vi "Init Hardware.vi"(8 "error in (no error)":errorcluster, 11 "Micron sm Digitizer in":refnum<class "Micron sm Digitizer.lvclass">) -> (0 "error out":errorcluster, 3 "Micron sm Digitizer out":refnum<class "Micron sm Digitizer.lvclass">)   [LabVIEW 2024, in "Micron sm Digitizer.lvclass"]
uses:
  Micron sm Digitizer.lvclass
  C:/Git/NHMFL_Core/Libraries/Instruments/VISA Instrument/VISA Instrument.lvclass
  C:/Git/NHMFL_Core/Libraries/Instruments/Instrument Driver/Instrument Driver.lvclass
  VISA Instrument/VISA Instrument.lvclass/VISA Instrument.ctl
  Instrument Driver/Instrument Driver.lvclass/Instrument Driver.ctl
  VISA Instrument/Read VISA resource.vi
  Instrument Driver/Read Cycle period.vi
  VISA Instrument/Write VISA resource.vi
  Micron Optics sm130/Micron Optics sm130.lvlib
panel:
  out "Rate":i32
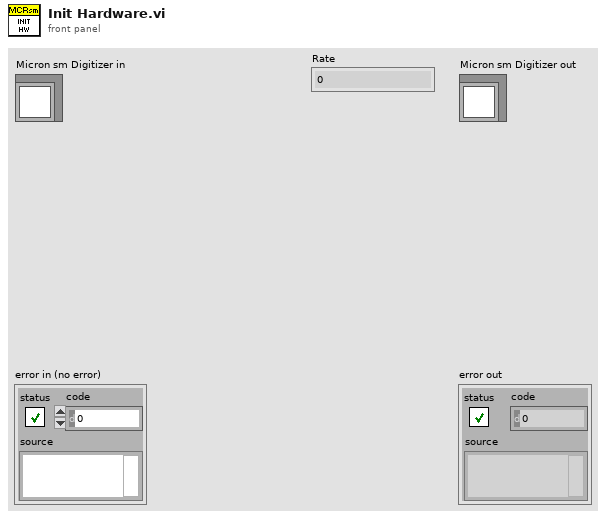
[diagram p1: front panel]
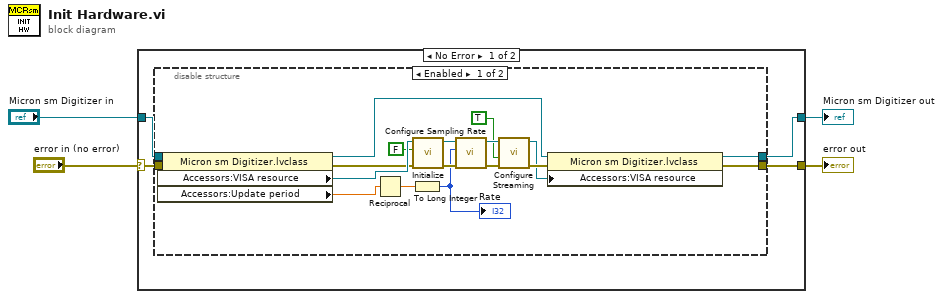
[diagram p0: block diagram]
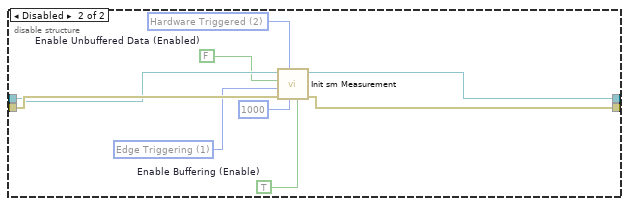
[diagram p2: hidden frame]
diagram:
  n1 = case shown="No Error" "error in (no error)" {
    selector: "error in (no error)" -> [w5 w36]
    tunnel: "Micron sm Digitizer in" -> [w8 w37]
    tunnel: [w7 w36] -> w3
    tunnel: [w6 w37] -> w2
    frame No Error {
      n2 = disable-structure shown="Enabled" {
        disable-tunnel: w8 -> [w26 w33]
        disable-tunnel: [w12 w34] -> w7
        disable-tunnel: [w11 w32] -> w6
        disable-tunnel: w5 -> [w10 w35]
        frame Enabled {
          n3 = property class="Micron sm Digitizer.lvclass"(reference=w26, error in=w10) -> (reference out=w15:refnum<class "Micron sm Digitizer.lvclass">, error out=w24:errorcluster, "Accessors:VISA resource"=w25:refnum<visa-resource-name>, "Accessors:Update period"=w21:dbl)
          n4 = Reciprocal(x=w21) -> (1/x=w20:dbl)
          n5 = To Long Integer(number=w20) -> (32bit integer=w19:i32)
          "Rate" <- w19
          n6 = call "Initialize.vi"("error in (no error)"=w24, "ID Query (True)"=FALSE, "VISA resource name"=w25) -> ("error out"=w23:errorcluster, "VISA resource name out"=w22:refnum<visa-resource-name>)  [unwired: 7 in]
          n7 = call "Configure Sampling Rate.vi"("error in (no error)"=w23, "Sample Rate (1000 Hz)"=w19, "VISA resource name"=w22) -> ("error out"=w17:errorcluster, "VISA resource name out"=w18:refnum<visa-resource-name>)  [unwired: 7 in]
          n8 = call "Configure Streaming.vi"("error in (no error)"=w17, "Enable Streaming (Enable)"=TRUE, "VISA resource name"=w18) -> ("error out"=w14:errorcluster, "VISA resource name out"=w13:refnum<visa-resource-name>)  [unwired: 7 in]
          n9 = property class="Micron sm Digitizer.lvclass"(reference=w15, error in=w14, "Accessors:VISA resource"=w13) -> (reference out=w11:refnum<class "Micron sm Digitizer.lvclass">, error out=w12:errorcluster)
        }
        frame Disabled {
          w28 = u16 2 items=["Untriggered", "Software Triggered", "Hardware Triggered"] ("Trigger Type (0:Untriggered)")
          w29 = FALSE  # Enable Unbuffered Data (Enabled)
          w30 = TRUE  # Enable Buffering (Enable)
          w31 = u16 1 items=["Number of Acquisitions", "Edge Triggering"] ("Trigger Stop Condition (1:Edge Triggering)")
          n10 = call-dynamic "Init sm Measurement.vi"("Enable Buffering (Enable)"=w30, "Number of Acquisitions (100)"=1000, "Trigger Type (0:Untriggered)"=w28, "error in (no error)"=w35, "Trigger Stop Condition (1:Edge Triggering)"=w31, "Enable Unbuffered Data (Enabled)"=w29, "Micron sm Digitizer in"=w33) -> ("error out"=w34:errorcluster, "Micron sm Digitizer out"=w32:refnum<class "Micron sm Digitizer.lvclass">)  [unwired: 2 in, 1 out]
        }
      }
    }
    frame Error {
    }
  }
  "error out" <- w3
  "Micron sm Digitizer out" <- w2
